vi "Event Wait Raw.vi"(8 "error in (no error)":errorcluster, 11 "Event DVR in":refnum<data-value>) -> (0 "error out":errorcluster, 2 "Raw data out":i8[](array[numeric]), 3 "Event DVR out":refnum<data-value>)   [LabVIEW 2012]
doc: "Get data received as a raw buffer."
uses:
  <vilib>/MDSplus/Classes/Event_Class/Event.lvclass
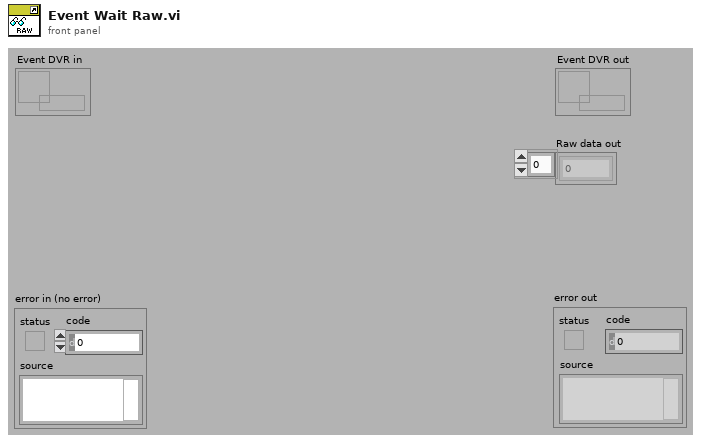
[diagram p1: front panel]
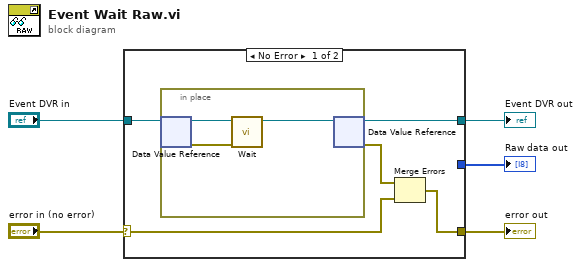
[diagram p0: block diagram]
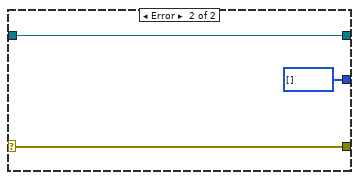
[diagram p2: hidden frame]
diagram:
  n1 = case shown="No Error" "error in (no error)" {
    selector: "error in (no error)" -> [w9 w16]
    tunnel: "Event DVR in" -> [w10 w15]
    tunnel: [w7 w16] -> w5
    tunnel: [w6 w15] -> w2
    tunnel: [_ i8[] [] ("Raw out")] -> w1
    frame No Error {
      n2 = in-place {
        n3 = in-place-dvr #1(w10) -> (w13:refnum<class "Event.lvclass">, w11:errorcluster)
        n4 = call-dynamic "Wait.vi"("error in (no error)"=w11, "Event in"=w13) -> ("Event out"=w12:refnum<class "Event.lvclass">)  [unwired: 7 in, 2 out]
        n5 = in-place-dvr #1(w12) -> (w6:refnum<data-value>, w8:errorcluster)
      }
      n6 = Merge Errors(w8, w9) -> (w7:errorcluster)  [unwired: 1 in]
    }
    frame Error {
    }
  }
  "error out" <- w5
  "Event DVR out" <- w2
  "Raw data out" <- w1
